vi "kethley_INI.vi"(9 "Function (0: Volts) in":u16(ring) items=["Volts", "Current", "Resistance"], 10 "Source Compaliance":dbl=1e-06, 11 "VISA Refnum in":refnum<visa-resource-name>) -> (1 "VISA resource name out":refnum<visa-resource-name>)   [LabVIEW 2021]
uses:
  <instrlib>/Keithley 2450/Keithley 2450.lvlib
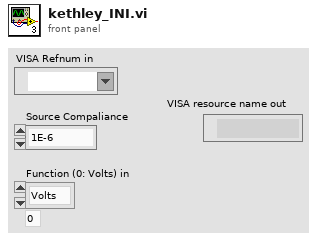
[diagram p1: front panel]
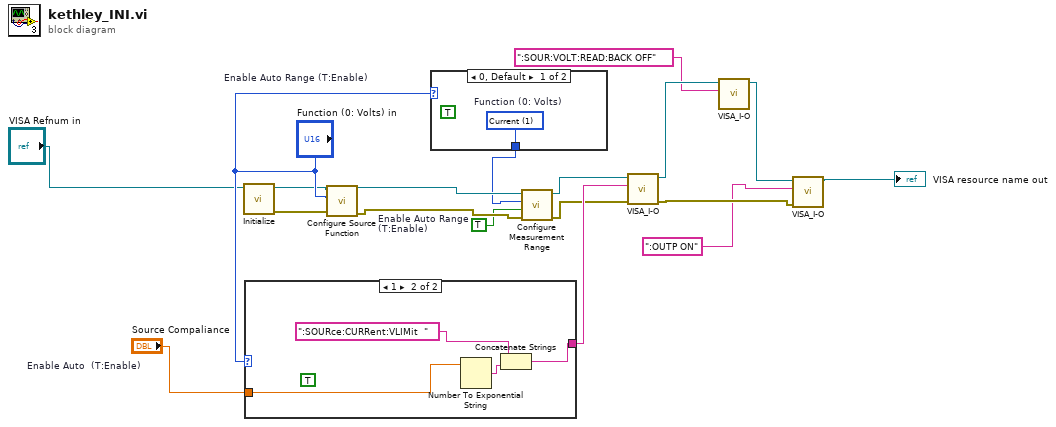
[diagram p0: block diagram]
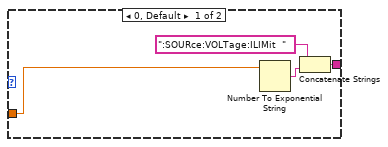
[diagram p2: hidden frame]
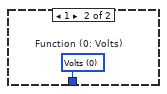
[diagram p3: hidden frame]
diagram:
  (unwired) TRUE  # Enable Auto  (T:Enable)
  w8 = TRUE  # Enable Auto Range (T:Enable)
  (unwired) TRUE  # Enable Auto Range (T:Enable)
  n1 = call <instrlib>:"Initialize.vi"("VISA resource name"="VISA Refnum in") -> ("error out"=w10:errorcluster, "VISA resource name out"=w6:refnum<visa-resource-name>)  [unwired: 9 in]
  n2 = case shown="1" "Function (0: Volts) in" {
    tunnel: [w20 w25] -> w14
    tunnel: "Source Compaliance" -> [w19 w23]
    frame 0, Default {
      n3 = Number To Exponential String(number=w19) -> (E-format string=w22:string)  [unwired: 3 in]
      n4 = Concatenate Strings(":SOURce:VOLTage:ILIMit  " ("write buffer (\"\")"), w22) -> (w20:string)
    }
    frame 1 {
      n5 = Number To Exponential String(number=w23) -> (E-format string=w26:string)  [unwired: 3 in]
      n6 = Concatenate Strings(":SOURce:CURRent:VLIMit  " ("write buffer (\"\")"), w26) -> (w25:string)
    }
  }
  n7 = call <instrlib>:"Configure Source Function.vi"("error in (no error)"=w10, "Function (0: Volts)"="Function (0: Volts) in", "VISA resource name"=w6) -> ("error out"=w12:errorcluster, "VISA resource name out"=w13:refnum<visa-resource-name>)  [unwired: 7 in]
  n8 = case shown="0, Default" "Function (0: Volts) in" {
    tunnel: [w27 w28] -> w7
    frame 0, Default {
      w27 = u16 1 items=["Volts", "Current", "Resistance"]  # Function (0: Volts)
    }
    frame 1 {
      w28 = u16 0 items=["Volts", "Current", "Resistance"]  # Function (0: Volts)
    }
  }
  n9 = call <instrlib>:"Configure Measurement Range.vi"("error in (no error)"=w12, "Enable Auto Range (T:Enable)"=w8, "Function (0: Volts)"=w7, "VISA resource name"=w13) -> ("error out"=w11:errorcluster, "VISA resource name out"=w9:refnum<visa-resource-name>)  [unwired: 6 in]
  n10 = call "VISA_I-O.vi"("error in (no error)"=w11, "write buffer"=w14, "VISA resource name"=w9) -> ("error out"=w17:errorcluster, "VISA resource name out"=w3:refnum<visa-resource-name>)  [unwired: 6 in, 1 out]
  n11 = call "VISA_I-O.vi"("write buffer"=":SOUR:VOLT:READ:BACK OFF" ("write buffer (\"\")"), "VISA resource name"=w3) -> ("VISA resource name out"=w2:refnum<visa-resource-name>)  [unwired: 7 in, 2 out]
  n12 = call "VISA_I-O.vi"("error in (no error)"=w17, "write buffer"=":OUTP ON" ("write buffer (\"\")"), "VISA resource name"=w2) -> ("VISA resource name out"=→"VISA resource name out":refnum<visa-resource-name>)  [unwired: 6 in, 2 out]
